vi "CalcWL.vi"(2 "Spectra":dbl[](array[numeric]), 3 "Lambda":dbl[](array[numeric])) -> (0 "CWl":dbl, 1 "Peak WL":dbl)   [LabVIEW 2012]
panel:
  out "FWHM Raw":dbl
  out "Spectral Results":T1
  out "Left Band":cluster{dbl[], dbl[]}
  out "Right Band":cluster{dbl[], dbl[]}
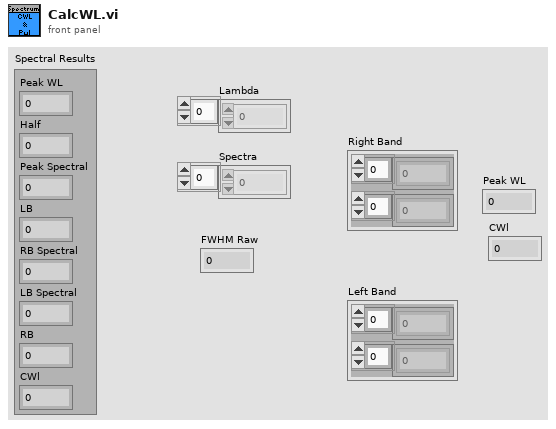
[diagram p1: front panel]
types:
  T1 = cluster{"Peak WL":dbl, "Half":dbl, "Peak Spectral":dbl, "LB":dbl, "RB Spectral":dbl, "LB Spectral":dbl, "RB":dbl, "CWl":dbl}
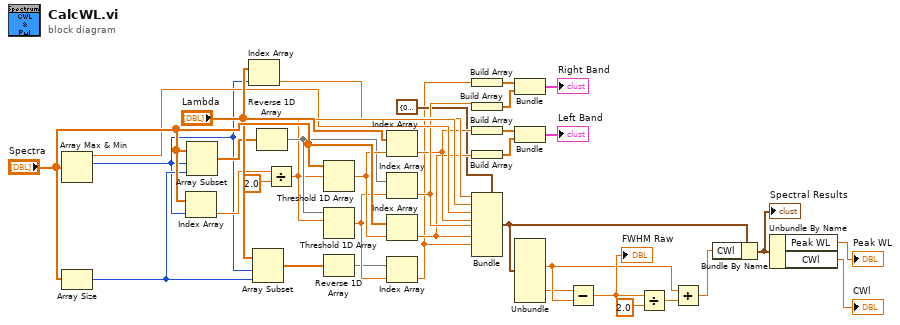
[diagram p0: block diagram]
diagram:
  n1 = Array Max & Min(array="Spectra") -> (max value=w18:dbl, max index (indices)=w17:i32)  [unwired: 2 out]
  n2 = Array Size(array="Spectra") -> (size(s)=w28:i32)
  n3 = Index Array(array="Spectra", index=w17) -> (element=w27:dbl)
  n4 = Array Subset(array="Spectra", index=w17, length=w28) -> (w29:dbl[])
  n5 = Index Array "Index Array"(array="Lambda", index=w17) -> (element=w16:dbl)
  n6 = Array Subset(array="Lambda", index=w17, length=w28) -> (w30:dbl[])
  n7 = Reverse 1D Array(array=w29) -> (reversed array=w33:dbl[])
  n8 = Divide(x=w27, y=2.0) -> (x/y=w19:dbl)
  n9 = Threshold 1D Array(2:w19, 3:"Spectra") -> (0:w34:dbl)  [unwired: 1 in]
  n10 = Threshold 1D Array(2:w19, 3:w33) -> (0:w32:dbl)  [unwired: 1 in]
  n11 = Reverse 1D Array(array=w30) -> (reversed array=w31:dbl[])
  n12 = Index Array(array="Lambda", index=w34) -> (element=w14:dbl)
  n13 = Index Array(array=w33, index=w32) -> (element=w15:dbl)
  n14 = Index Array(array="Spectra", index=w34) -> (element=w13:dbl)
  n15 = Index Array(array=w31, index=w32) -> (element=w11:dbl)
  n16 = Build Array(w11) -> (w25:dbl[])
  n17 = Build Array(w15) -> (w24:dbl[])
  n18 = Build Array(w14) -> (w22:dbl[])
  n19 = Build Array(w13) -> (w21:dbl[])
  n20 = Bundle(cluster=T1 {"Peak WL"=0.0, "Half"=0.0, "Peak Spectral"=0.0, "LB"=0.0, "RB Spectral"=0.0, "LB Spectral"=0.0, "RB"=0.0, "CWl"=0.0} ("Spectral Results"), "Peak WL"=w16, "Half"=w19, "Peak Spectral"=w18, "LB"=w14, "RB Spectral"=w15, "LB Spectral"=w13, "RB"=w11) -> (w5:T1)  [unwired: 1 in]
  n21 = Bundle(w25, w24) -> (→"Right Band":cluster{dbl[], dbl[]})  [unwired: 1 in]
  n22 = Bundle(w22, w21) -> (→"Left Band":cluster{dbl[], dbl[]})  [unwired: 1 in]
  n23 = Unbundle(w5) -> ("LB"=w7:dbl, "RB"=w6:dbl)  [unwired: 6 out]
  n24 = Subtract(x=w6, y=w7) -> (x-y=w10:dbl)
  "FWHM Raw" <- w10
  n25 = Divide(x=w10, y=2.0) -> (x/y=w8:dbl)
  n26 = Add(x=w7, y=w8) -> (x+y=w4:dbl)
  n27 = Bundle By Name(cluster=w5, "CWl"=w4) -> (w3:T1)
  "Spectral Results" <- w3
  n28 = Unbundle By Name(w3) -> ("Peak WL"=→"Peak WL":dbl, "CWl"=→"CWl":dbl)
